vi "LvMPDC_Global_Setting.vi"() -> ()   [LabVIEW 2012]
panel:
  in  "Port":u16
  in  "Server":string
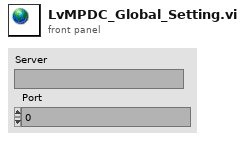
[diagram p1: front panel]
diagram:
